vi "TCP-error-string.vi"(8 "error in (no error)":errorcluster, 10 "Retun code":string) -> (0 "error out":errorcluster)   [LabVIEW 2013, in "MaterialCharacterization.lvlib" / "MC-SM1000.lvclass"]
doc: "Verified if the return string contains at least the \nexpected string. Case insensitive."
uses:
  MC-SM1000.lvclass
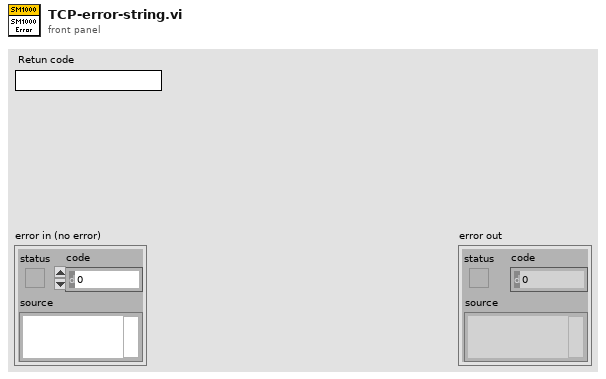
[diagram p1: front panel]
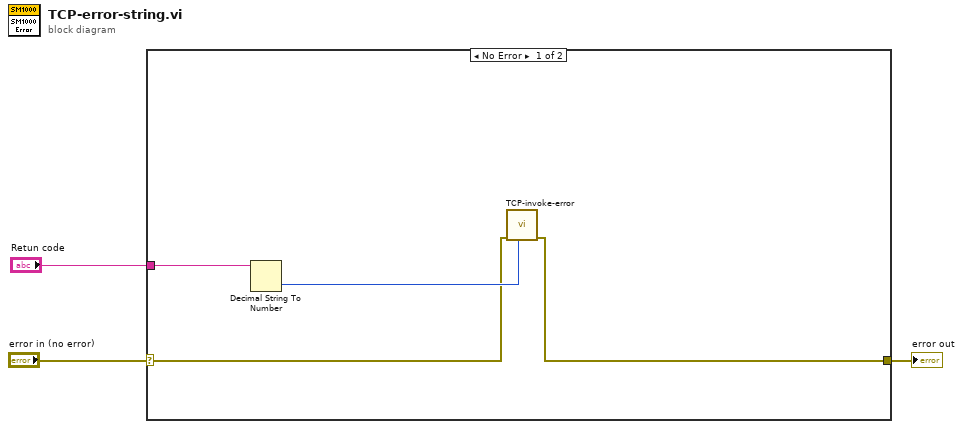
[diagram p0: block diagram]
diagram:
  n1 = case shown="No Error" "error in (no error)" {
    selector: "error in (no error)" -> [w5 w8]
    tunnel: [w4 w8] -> w2
    tunnel: "Retun code" -> [w7 _]
    frame No Error {
      n2 = Decimal String To Number(string=w7) -> (number=w6:i32)  [unwired: 2 in, 1 out]
      n3 = call "TCP-invoke-error.vi"("Return-code"=w6, "error in (no error)"=w5) -> ("error out"=w4:errorcluster)  [unwired: 9 in]
    }
    frame Error {
    }
  }
  "error out" <- w2
